vi "runTestScenario.vi"(8 "error in (no error)":errorcluster, 11 "VrefTest in":refnum<class "VrefTest.lvclass">) -> (0 "error out":errorcluster, 2 "TestExecution":T1, 3 "VrefTest out":refnum<class "VrefTest.lvclass">)   [LabVIEW 2015, in "VrefTest.lvclass"]
uses:
  VrefTest.lvclass
  Typedefs/TestExecution.ctl
  Typedefs/WriteDataFileInput.ctl
  Typedefs/TestScenarioTypes.ctl
  Typedefs/WriteLogMessageInput.ctl
  Typedefs/PassFailTest.ctl
  VrefTest.lvclass/VrefTest.ctl
  Model/TestLog/ITestLog/ITestLog.lvclass
  Typedefs/ILCBTTypedefs.lvlib
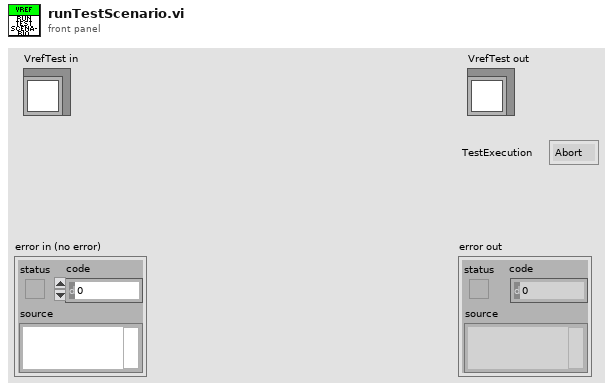
[diagram p1: front panel]
types:
  T1 = typedef "ILCBTTypedefs.lvlib/TestExecution.ctl" = enum16{"Abort", "Continue"}
  T2 = typedef "ILCBTTypedefs.lvlib/WriteLogMessageInput.ctl" = cluster{"Test Scenario":T3, "Description":string, "Actual Value":string, "Data File":string, "Result":T4}
  T3 = typedef "ILCBTTypedefs.lvlib/TestScenarioTypes.ctl" = enum16{"+3.3VA Supply Test", "+3.3VD Supply Test", "+5VA Supply Test", "+5VD Supply Test", "Unique ID Test", "TEDS Status Test", "LIMSW1_TTL Low Test", "LIMSW1_TTL High Test", "LIMSW2_TTL Low Test", "LIMSW2_TTL High Test", "Tachometer Test", "SSR_TTL Low Test", "SSR_TTL High Test", "SM_CW Low Test", "SM_CW High Test", "SM_CCW Low Test", "SM_CCW High Test", "SM_GPI Low Test", "SM_GPI High Test", "CW Motion Without Limit Test", "CW Motion With Limit Test", "CW Motion With Limit Interruption Test", "CW Motion on CCW Limit Test", "CCW Motion Without Limit Test", "CCW Motion With Limit Test", "CCW Motion With Limit Interruption Test", "CCW Motion on CW Limit Test", "RS232-TXD Low Test", "RS232-TXD High Test", "RS232-RTS Low Test", "RS232-RTS High Test", "RS232-RXD Low Test", "RS232-RXD High Test", "RS232-CTS Low Test", "RS232-CTS High Test", "Out_SS Low Test", "Out_SS High Test", "Out_SDI Low Test", "Out_SDI High Test", "Out_SCLK Low Test", "Out_SCLK High Test", "Reset Low Test", "Reset High Test", "1 Channel ADC Test", "3 Channel ADC Test", "5 Channel ADC Test", "Vref Test", "ROT Test", "DAC1 Test", "DAC2 Test", "DAC3 Test", "DAC4 Test", "BIAS Test", "EXC1 Test", "EXC2 Test", "EXC3 Test", "EXC4 Test"}
  T4 = typedef "ILCBTTypedefs.lvlib/PassFailTest.ctl" = enum16{"Fail", "Pass", "NA"}
  T5 = typedef "ILCBTTypedefs.lvlib/WriteDataFileInput.ctl" = cluster{"Test Scenario":T3, "File Name":string, "Output":dbl[]}
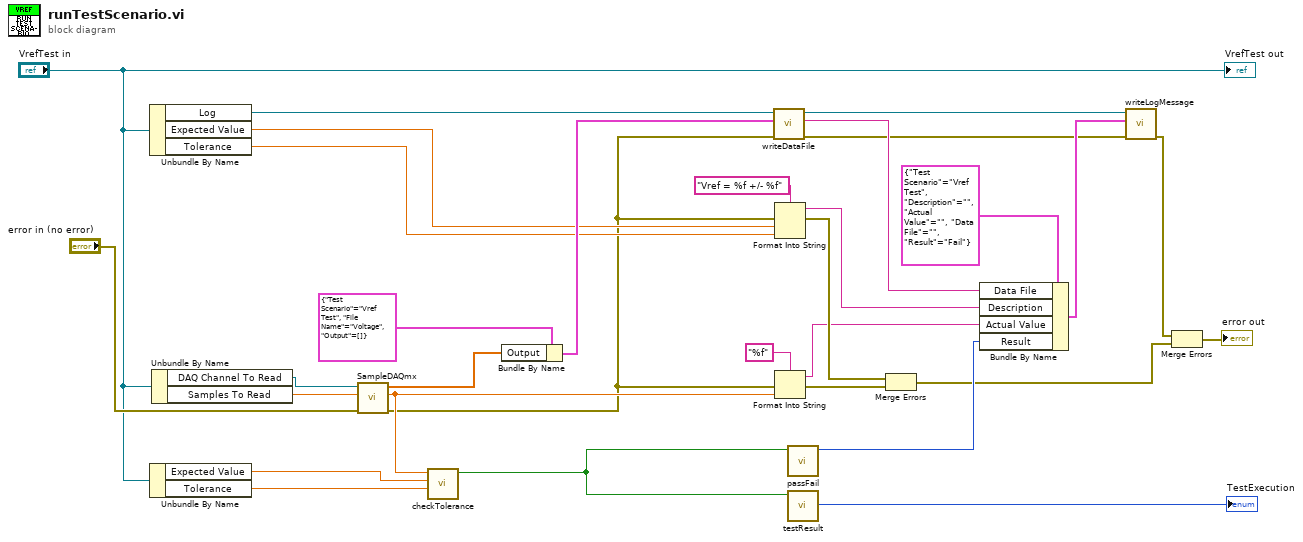
[diagram p0: block diagram]
diagram:
  n1 = Unbundle By Name("VrefTest in") -> ("Log"=w30:refnum<class "ITestLog.lvclass">, "Expected Value"=w14:dbl[unit], "Tolerance"=w13:dbl[unit])
  n2 = Unbundle By Name("VrefTest in") -> ("Expected Value"=w18:dbl[unit], "Tolerance"=w17:dbl[unit])
  n3 = Unbundle By Name("VrefTest in") -> ("DAQ Channel To Read"=w22:refnum<k21>, "Samples To Read"=w21:dbl)
  n4 = call "SampleDAQmx.vi"("error in (no error)"="error in (no error)", "Samples To Read"=w21, "DAQ Channel To Read"=w22) -> ("error out"=w12:errorcluster, "Average"=w15:dbl, "Samples"=w29:dbl[])  [unwired: 6 in]
  n5 = call "checkTolerance.vi"("Tolerance"=w17, "Expected Value"=w18, "Average"=w15) -> ("Boolean"=w16:bool)  [unwired: 8 in]
  n6 = Bundle By Name(cluster=T5 {"Test Scenario"=enum."Vref Test", "File Name"="Voltage", "Output"=[]} ("WriteDataFileInput"), "Output"=w29) -> (w19:T5)
  n7 = call-dynamic "writeDataFile.vi"("error in (no error)"=w12, "WriteDataFileInput"=w19, "ITestLog in"=w30) -> ("error out"=w9:errorcluster, "Relative Path"=w11:string, "ITestLog out"=w24:refnum<class "ITestLog.lvclass">)  [unwired: 6 in]
  n8 = Format Into String(format string="Vref = %f +/- %f", error in=w12, w14, w13) -> (resulting string=w10:string, error out=w8:errorcluster)  [unwired: 1 in]
  n9 = Format Into String(format string="%f", error in=w12, w15) -> (resulting string=w3:string, error out=w7:errorcluster)  [unwired: 1 in]
  n10 = call "passFail.vi"("Boolean"=w16) -> ("Result"=w25:T4)  [unwired: 10 in]
  n11 = call "testResult.vi"("Boolean"=w16) -> ("TestExecution"=→"TestExecution":T1)  [unwired: 10 in]
  n12 = Merge Errors(w8, w7) -> (w4:errorcluster)
  n13 = Bundle By Name(cluster=T2 {"Test Scenario"=enum."Vref Test", "Description"="", "Actual Value"="", "Data File"="", "Result"=enum."Fail"} ("WriteLogMessageInput"), "Data File"=w11, "Description"=w10, "Actual Value"=w3, "Result"=w25) -> (w23:T2)
  n14 = call-dynamic "writeLogMessage.vi"("error in (no error)"=w9, "WriteLogMessageInput"=w23, "ITestLog in"=w24) -> ("error out"=w5:errorcluster)  [unwired: 7 in, 1 out]
  n15 = Merge Errors(w5, w4) -> (→"error out":errorcluster)
  "VrefTest out" <- "VrefTest in"
